vi "svReadSerialAndGetLine.vi"(8 "error in (no error)":errorcluster, 11 "VISA Refnum in":refnum<visa-resource-name>) -> (0 "error out":errorcluster, 2 "One data line":string, 3 "VISA Refnum out":refnum<visa-resource-name>)   [LabVIEW 2021]
uses:
  enumFGVstringBuffer.ctl
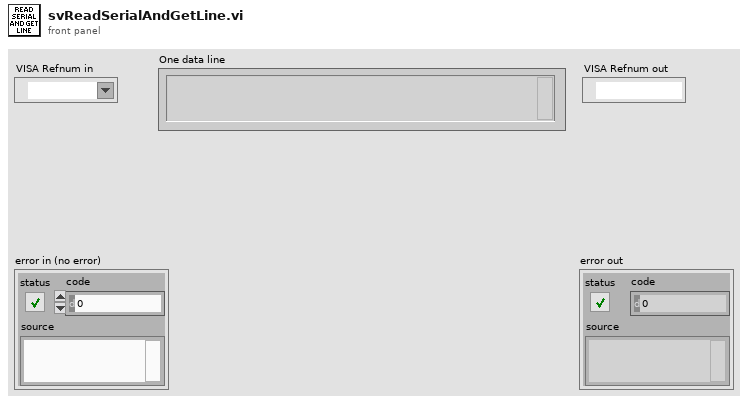
[diagram p1: front panel]
types:
  T1 = typedef "enumFGVstringBuffer.ctl" = enum16{"Init", "Write", "Read"}
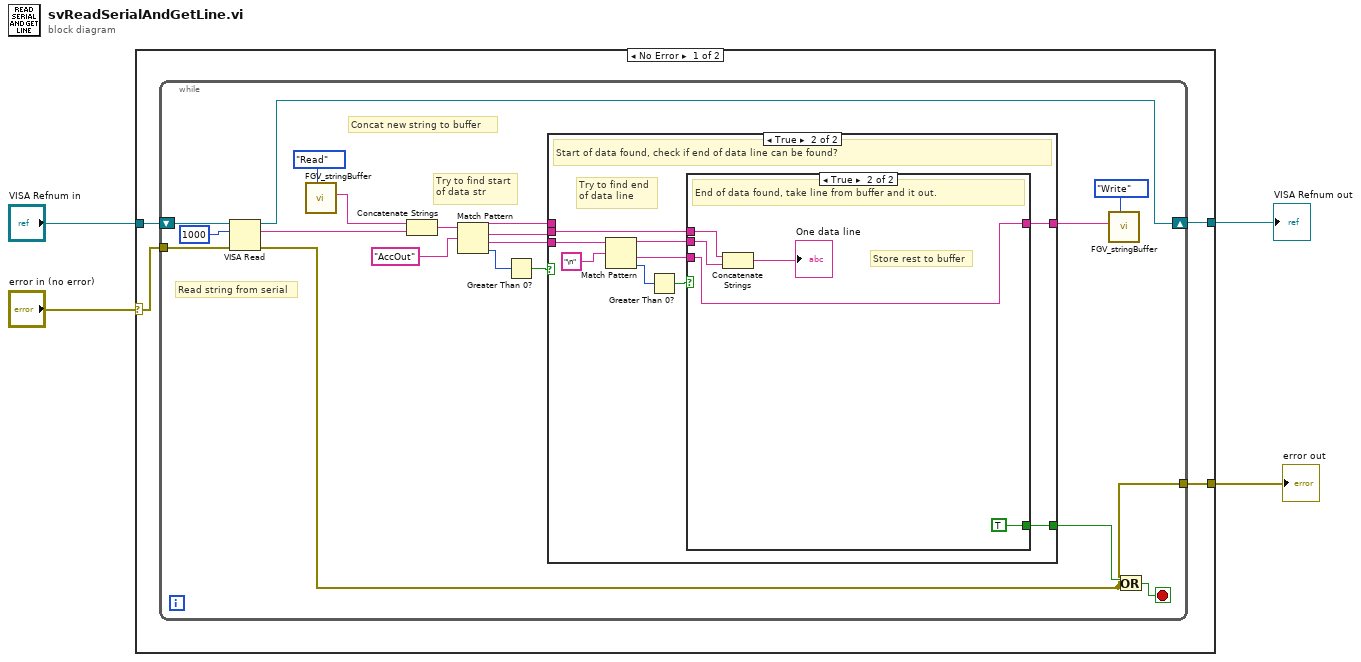
[diagram p0: block diagram]
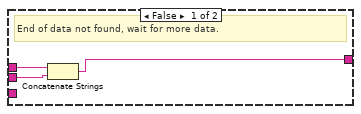
[diagram p3: hidden frame]
diagram:
  n1 = case shown="No Error" "error in (no error)" {
    selector: "error in (no error)" -> [w6 w46]
    tunnel: [w8 w47] -> w4
    tunnel: "VISA Refnum in" -> [w7 w47]
    tunnel: [w5 w46] -> w1
    frame No Error {
      n2 = while {
        tunnel: w6 -> [w26]
        shift-right: [w12] -> w8
        shift-left: w7 -> [w25]
        tunnel: [w9] -> w5
        stop <- w11 stop-if-true
        # "Concat new string to buffer"
        # "Try to find start\nof data str"
        # "Read string from serial"
        n3 = VISA Read(VISA resource name=w25, byte count=u32 1000 ("Read Count"), error in (no error)=w26) -> (VISA resource name out=w12:refnum<visa-resource-name>, read buffer=w20:string, error out=w9:errorcluster)  [unwired: 1 out]
        n4 = call "FGV_stringBuffer.vi"("Enum"=enumFGVstringBuffer."Read") -> ("String Out"=w19:string)  [unwired: 9 in, 1 out]
        n5 = Concatenate Strings(w19, w20) -> (w21:string)
        n6 = Match Pattern(string=w21, regular expression="AccOut" ("input string")) -> (before substring=w15:string, match substring=w16:string, after substring=w17:string, offset past match=w23:i32)  [unwired: 1 in]
        n7 = Greater Than 0?(x=w23) -> (x > 0?=w18:bool)
        n8 = case shown="True" w18 {
          tunnel: w17 -> [_ w37]
          tunnel: [w28 w33] -> w13
          tunnel: w15 -> [w28 _]
          tunnel: w16 -> [_ w32]
          tunnel: [_ w29] -> w10
          frame False {
            # "Start of data not found - wait for more data in buffer."
          }
          frame True {
            # "Try to find end\nof data line"
            # "Start of data found, check if end of data line can be found?"
            n9 = Match Pattern(string=w37, regular expression="\n" ("input string")) -> (before substring=w36:string, after substring=w31:string, offset past match=w35:i32)  [unwired: 1 in, 1 out]
            n10 = Greater Than 0?(x=w35) -> (x > 0?=w34:bool)
            n11 = case shown="True" w34 {
              tunnel: w36 -> [w40 w43]
              tunnel: [w39 w42] -> w33
              tunnel: w31 -> [_ w42]
              tunnel: w32 -> [w38 w44]
              tunnel: [_ TRUE ("x .or. y?")] -> w29
              frame False {
                # "End of data not found, wait for more data."
                n12 = Concatenate Strings(w38, w40) -> (w39:string)
              }
              frame True {
                # "Store rest to buffer"
                # "End of data found, take line from buffer and it out."
                n13 = Concatenate Strings(w44, w43) -> (→"One data line":string)
              }
            }
          }
        }
        n14 = call "FGV_stringBuffer.vi"("Enum"=enumFGVstringBuffer."Write", "String In"=w13) -> ()  [unwired: 8 in, 2 out]
        n15 = Or(x=w10, y=w9) -> (x .or. y?=w11:bool)
      }
    }
    frame Error {
    }
  }
  "VISA Refnum out" <- w4
  "error out" <- w1
